vi "Test.vi"() -> ()   [LabVIEW 2014]
uses:
  SPIBus0/Node/Controls/NodeResources FIFOs.ctl
  <vilib>/rvi/Emulation/niFpgaGetClockAttributes.vi
  <vilib>/rvi/Emulation/niFpgaSctlEmulationGetInTimedLoop.vi
  <vilib>/rvi/Emulation/niFpgaEmulationReportErrorSimple.vi
  <vilib>/rvi/Emulation/niFpgaCriticalErrorInLSC.vi
  SPIBus0/IO Node Logic Template_SPIBus0.lvlib
panel:
  out "Numeric":i32
  out "Received Data":u64
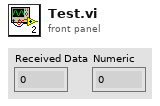
[diagram p1: front panel]
types:
  T1 = typedef "IO Node Logic Template_SPIBus0.lvlib/NodeResources FIFOs.ctl" = cluster{"SendCmdFIFO":refnum<k21>, "ReceiveDataFIFO":refnum<k21>}
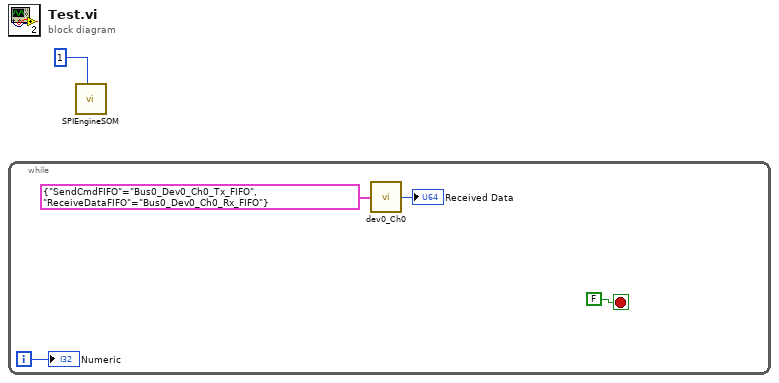
[diagram p0: block diagram]
diagram:
  n1 = while {
    i -> [w2]
    stop <- FALSE stop-if-true
    n2 = call "dev0_Ch0.vi"("FIFOs: I/O Node"=T1 {"SendCmdFIFO"="Bus0_Dev0_Ch0_Tx_FIFO", "ReceiveDataFIFO"="Bus0_Dev0_Ch0_Rx_FIFO"}) -> ("Received Data"=→"Received Data":u64)  [unwired: 14 in]
    "Numeric" <- w2
  }
  n3 = call "SPIEngineSOM.vi"("NumNodes"=u8 1) -> ()  [unwired: 11 in]
